vi "waveform_chart.vi"() -> ()   [LabVIEW 2022 SP3]
panel:
  out "Waveform Graph":dbl[](graph)
  out "Waveform Chart":dbl[](graph)
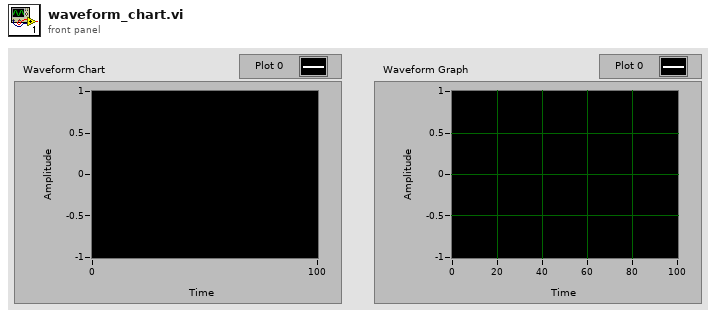
[diagram p1: front panel]
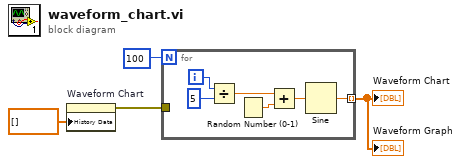
[diagram p0: block diagram]
diagram:
  n1 = property on="Waveform Chart" class="WFChart (严格)"("History Data"=dbl[] []) -> (error out=w2:errorcluster)  [unwired: 2 in, 1 out]
  n2 = for {
    N: 100 -> [_]
    tunnel: [w5] -> w1 mode=indexing
    tunnel: w2 -> [_]
    i -> [w10]
    n3 = Divide(x=w10, y=5) -> (x/y=w7:dbl)
    n4 = Random Number (0-1)() -> (number: 0 to 1=w8:dbl)
    n5 = Add(x=w7, y=w8) -> (x+y=w6:dbl)
    n6 = Sine(x=w6) -> (sin(x)=w5:dbl)
  }
  "Waveform Graph" <- w1
  "Waveform Chart" <- w1
